vi "Vision Align.vi"() -> (3 "YawAdjustment":dbl)   [LabVIEW 2019]
uses:
  <vilib>/Rock Robotics/Network Tables/NT Read Numeric Array.vi
  <vilib>/Rock Robotics/Network Tables/NT Write Boolean.vi
  Robot Global Data.vi
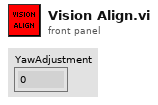
[diagram p1: front panel]
types:
  T1 = cluster{"Yaw":dbl, "Roll":dbl, "Pitch":dbl, "Heading":dbl, "Fused Heading":dbl}
  T2 = typedef "WPI_EncoderDevRef.ctl" = cluster{"DevStatus":errorcluster, "EncoderIndex":T3, "CounterIndex":T4, "DistancePerCount":dbl, "Decoding Type":T5}
  T3 = typedef "FPGA_EncoderIdx.ctl" = enum8{"Enc 0", "Enc 1", "Enc 2", "Enc 3", "Enc 4", "Enc 5", "Enc 6", "Enc 7", "Invalid"}
  T4 = typedef "FPGA_CounterCtrSystemIndex.ctl" = enum8{"Ctr 0", "Ctr 1", "Ctr 2", "Ctr 3", "Ctr 4", "Ctr 5", "Ctr 6", "Ctr 7", "Invalid"}
  T5 = typedef "WPI_EncoderType.ctl" = enum16{"1x", "2x", "4x"}
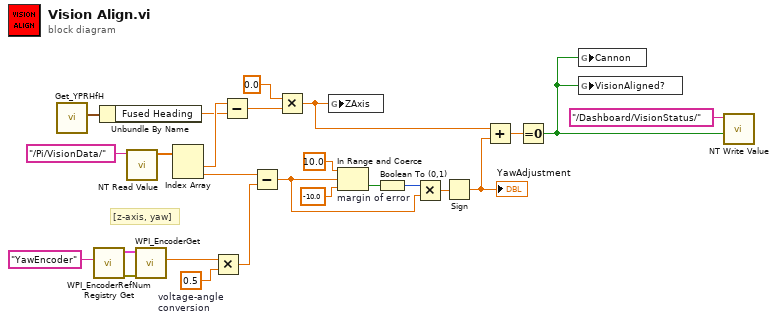
[diagram p0: block diagram]
diagram:
  w18 = 0.5  # voltage-angle conversion
  # "[z-axis, yaw]"
  n1 = call <vilib>:"Get_YPRHfH.vi"() -> ("YRPHfH"=w13:T1)  [unwired: 11 in]
  n2 = call <vilib>:"WPI_EncoderRefNum Registry Get.vi"("refnum name"="YawEncoder") -> ("error out"=w22:errorcluster, "EncoderDevRef"=w23:T2)  [unwired: 9 in]
  n3 = Unbundle By Name(w13) -> ("Fused Heading"=w11:dbl)
  n4 = call-poly <vilib>:"NT Read Value.vi"("Name"="/Pi/VisionData/") -> ("Numeric Array"=w24:dbl[])  [unwired: 9 in, 1 out]
  n5 = call <vilib>:"WPI_EncoderGet.vi"("error in (no error)"=w22, "EncoderDevRef"=w23) -> ("Distance"=w19:dbl)  [unwired: 4 in, 5 out]
  n6 = Index Array(array=w24) -> (element #1=w12:dbl, element #2=w20:dbl)  [unwired: 2 in]
  n7 = Multiply(x=w19, y=w18) -> (x*y=w17:dbl)
  n8 = Subtract(x=w12, y=w11) -> (x-y=w9:dbl)
  n9 = Subtract(x=w20, y=w17) -> (x-y=w3:dbl)
  n10 = Multiply(x=0.0, y=w9) -> (x*y=w10:dbl)
  n11 = global write "Robot Global Data.vi" "ZAxis"(w10) -> ()
  n12 = In Range and Coerce "margin of error"(upper limit=10.0, x=w3, lower limit=-10.0) -> (In Range?=w5:bool)  [unwired: 1 out]
  n13 = Boolean To (0,1)(Boolean=w5) -> (0, 1=w4:i16)
  n14 = Multiply(x=w4, y=w3) -> (x*y=w2:dbl)
  n15 = Sign(1:w2) -> (0:w1:dbl)
  "YawAdjustment" <- w1
  n16 = Add(x=w10, y=w1) -> (x+y=w15:dbl)
  n17 = Equal To 0?(x=w15) -> (x = 0?=w14:bool)
  n18 = global write "Robot Global Data.vi" "Cannon"(w14) -> ()
  n19 = global write "Robot Global Data.vi" "VisionAligned?"(w14) -> ()
  n20 = call-poly <vilib>:"NT Write Value.vi"("Boolean"=w14, "Name"="/Dashboard/VisionStatus/") -> ()  [unwired: 9 in, 1 out]
